vi "Open Pneumatics.vi"(9 "PCM CAN ID":u8) -> ()   [LabVIEW 2018]
uses:
  <vilib>/Rock Robotics/WPI/Solenoid/WPI_SolenoidChannel.ctl
  <vilib>/Rock Robotics/WPI/Solenoid/WPI_SolenoidValue.ctl
  <vilib>/Rock Robotics/WPI/Solenoid/WPI_SolenoidOpenDouble.vi
  <vilib>/Rock Robotics/WPI/Utilities/WPI_GetSetVariantRefNum.vi
  <vilib>/Rock Robotics/WPI/Solenoid/WPI_SolenoidSetEnum.vi
  <vilib>/Rock Robotics/WPI/Solenoid/WPI_SolenoidOpenSingle.vi
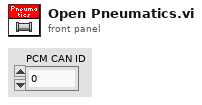
[diagram p1: front panel]
types:
  T1 = typedef "WPI_SolenoidValue.ctl" = enum16{"Off", "On", "Forward", "Reverse"}
  T2 = typedef "WPI_SolenoidChannel.ctl" = enum8{"Solenoid 0", "Solenoid 1", "Solenoid 2", "Solenoid 3", "Solenoid 4", "Solenoid 5", "Solenoid 6", "Solenoid 7", "Invalid"}
  T3 = typedef "WPI_SolenoidDevRef.ctl" = cluster{"DevStatus":errorcluster, "Pneumatics Control Module":u8, "Forward Solenoid Channel":T2, "Reverse Solenoid Channel":T2}
  T4 = typedef "WPI_CompressorDevRef.ctl" = cluster{"DevStatus":errorcluster, "Pneumatics Control Module":u8}
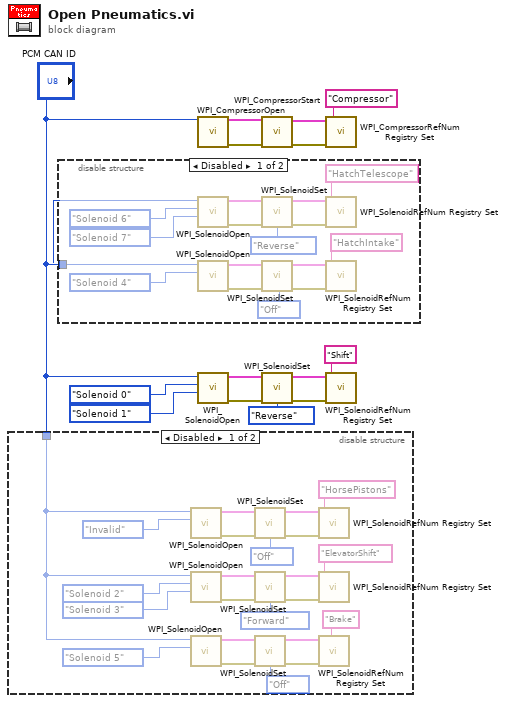
[diagram p0: block diagram]
diagram:
  n1 = disable-structure shown="Disabled" {
    disable-tunnel: "PCM CAN ID" -> [w15 _]
    frame Disabled {
      n2 = call-poly <vilib>:"WPI_SolenoidOpen.vi"("Solenoid Channel"=WPI_SolenoidChannel."Invalid", "Pneumatics Control Module (0)"=w15) -> ("error out"=w28:errorcluster, "SolenoidDevRef"=w31:T3)  [unwired: 8 in]
      n3 = call-poly <vilib>:"WPI_SolenoidOpen.vi"("Reverse Solenoid Channel"=WPI_SolenoidChannel."Solenoid 3", "Forward Solenoid Channel"=WPI_SolenoidChannel."Solenoid 2" ("Solenoid Channel"), "Pneumatics Control Module (0)"=w15) -> ("error out"=w26:errorcluster, "SolenoidDevRef"=w30:T3)  [unwired: 7 in]
      n4 = call-poly <vilib>:"WPI_SolenoidOpen.vi"("Solenoid Channel"=WPI_SolenoidChannel."Solenoid 5", "Pneumatics Control Module (0)"=w15) -> ("error out"=w19:errorcluster, "SolenoidDevRef"=w21:T3)  [unwired: 8 in]
      n5 = call-poly <vilib>:"WPI_SolenoidSet.vi"("error in (no error)"=w28, "Value"=WPI_SolenoidValue."Off", "SolenoidDevRef"=w31) -> ("error out"=w27:errorcluster, "SolenoidDevRef"=w32:T3)  [unwired: 7 in]
      n6 = call-poly <vilib>:"WPI_SolenoidSet.vi"("error in (no error)"=w26, "Value"=WPI_SolenoidValue."Forward", "SolenoidDevRef"=w30) -> ("error out"=w25:errorcluster, "SolenoidDevRef"=w29:T3)  [unwired: 7 in]
      n7 = call-poly <vilib>:"WPI_SolenoidSet.vi"("error in (no error)"=w19, "Value"=WPI_SolenoidValue."Off", "SolenoidDevRef"=w21) -> ("error out"=w18:errorcluster, "SolenoidDevRef"=w20:T3)  [unwired: 7 in]
      n8 = call <vilib>:"WPI_SolenoidRefNum Registry Set.vi"("error in (no error)"=w27, "refnum name"="HorsePistons", "SolenoidDevRef"=w32) -> ()  [unwired: 7 in, 2 out]
      n9 = call <vilib>:"WPI_SolenoidRefNum Registry Set.vi"("error in (no error)"=w25, "refnum name"="ElevatorShift", "SolenoidDevRef"=w29) -> ()  [unwired: 7 in, 2 out]
      n10 = call <vilib>:"WPI_SolenoidRefNum Registry Set.vi"("error in (no error)"=w18, "refnum name"="Brake", "SolenoidDevRef"=w20) -> ()  [unwired: 7 in, 2 out]
    }
    frame Enabled {
    }
  }
  n11 = disable-structure shown="Disabled" {
    disable-tunnel: "PCM CAN ID" -> [w39 _]
    frame Disabled {
      n12 = call-poly <vilib>:"WPI_SolenoidOpen.vi"("Reverse Solenoid Channel"=WPI_SolenoidChannel."Solenoid 7", "Forward Solenoid Channel"=WPI_SolenoidChannel."Solenoid 6", "Pneumatics Control Module (0)"=w39) -> ("error out"=w49:errorcluster, "SolenoidDevRef"=w45:T3)  [unwired: 7 in]
      n13 = call-poly <vilib>:"WPI_SolenoidOpen.vi"("Solenoid Channel"=WPI_SolenoidChannel."Solenoid 4", "Pneumatics Control Module (0)"=w39) -> ("error out"=w51:errorcluster, "SolenoidDevRef"=w48:T3)  [unwired: 8 in]
      n14 = call-poly <vilib>:"WPI_SolenoidSet.vi"("error in (no error)"=w49, "Value"=WPI_SolenoidValue."Reverse", "SolenoidDevRef"=w45) -> ("error out"=w50:errorcluster, "SolenoidDevRef"=w46:T3)  [unwired: 7 in]
      n15 = call-poly <vilib>:"WPI_SolenoidSet.vi"("error in (no error)"=w51, "Value"=WPI_SolenoidValue."Off", "SolenoidDevRef"=w48) -> ("error out"=w52:errorcluster, "SolenoidDevRef"=w47:T3)  [unwired: 7 in]
      n16 = call <vilib>:"WPI_SolenoidRefNum Registry Set.vi"("error in (no error)"=w50, "refnum name"="HatchTelescope", "SolenoidDevRef"=w46) -> ()  [unwired: 7 in, 2 out]
      n17 = call <vilib>:"WPI_SolenoidRefNum Registry Set.vi"("error in (no error)"=w52, "refnum name"="HatchIntake", "SolenoidDevRef"=w47) -> ()  [unwired: 7 in, 2 out]
    }
    frame Enabled {
    }
  }
  n18 = call <vilib>:"WPI_CompressorOpen.vi"("Pneumatics Control Module (0)"="PCM CAN ID") -> ("CompressorDevRef"=w12:T4, "error out"=w11:errorcluster)  [unwired: 13 in]
  n19 = call-poly <vilib>:"WPI_SolenoidOpen.vi"("Reverse Solenoid Channel"=WPI_SolenoidChannel."Solenoid 1", "Forward Solenoid Channel"=WPI_SolenoidChannel."Solenoid 0", "Pneumatics Control Module (0)"="PCM CAN ID") -> ("error out"=w4:errorcluster, "SolenoidDevRef"=w6:T3)  [unwired: 7 in]
  n20 = call <vilib>:"WPI_CompressorStart.vi"("error in (no error)"=w11, "CompressorDevRef"=w12) -> ("error out"=w14:errorcluster, "CompressorDevRef"=w13:T4)  [unwired: 8 in]
  n21 = call-poly <vilib>:"WPI_SolenoidSet.vi"("error in (no error)"=w4, "Value"=WPI_SolenoidValue."Reverse", "SolenoidDevRef"=w6) -> ("error out"=w3:errorcluster, "SolenoidDevRef"=w5:T3)  [unwired: 7 in]
  n22 = call <vilib>:"WPI_CompressorRefNum Registry Set.vi"("error in (no error)"=w14, "refnum name"="Compressor", "CompressorDevRef"=w13) -> ()  [unwired: 7 in, 2 out]
  n23 = call <vilib>:"WPI_SolenoidRefNum Registry Set.vi"("error in (no error)"=w3, "refnum name"="Shift", "SolenoidDevRef"=w5) -> ()  [unwired: 7 in, 2 out]
